vi "Initial AO Voltage.vi"(8 "error in":errorcluster, 11 "AO Properties":T1) -> (0 "error out":errorcluster, 3 "DAQ Ref out":refnum<k21>)   [LabVIEW 2021, in "DAQ Analog InOut Engine.lvlib"]
uses:
  DAQ Analog InOut Engine.lvlib
  AO Properties.ctl
  System Explorer/Types/Output Channel Parameters.ctl
  <vilib>/DAQmx/create/channels.llb/DAQmx Create Channel (AO-Voltage-Basic).vi
  System Explorer/DAQ Analog InOut System Explorer.lvlib
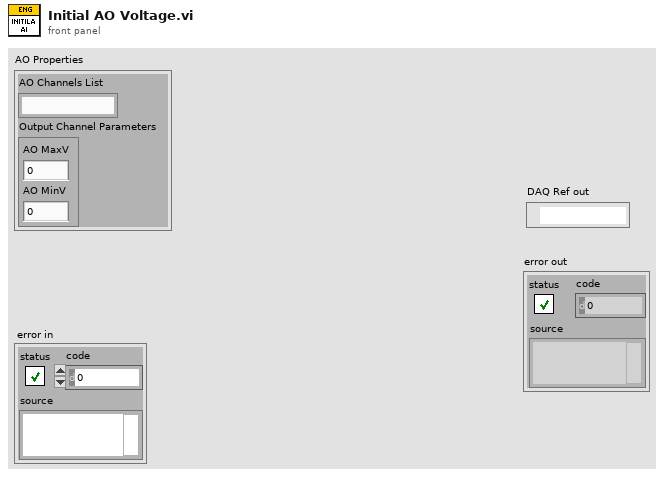
[diagram p1: front panel]
types:
  T1 = typedef "DAQ Analog InOut Engine.lvlib/AO Properties.ctl" = cluster{"AO Channels List":string, "Output Channel Parameters":T2}
  T2 = typedef "DAQ Analog InOut System Explorer.lvlib/Output Channel Parameters.ctl" = cluster{"AO MaxV":dbl, "AO MinV":dbl}
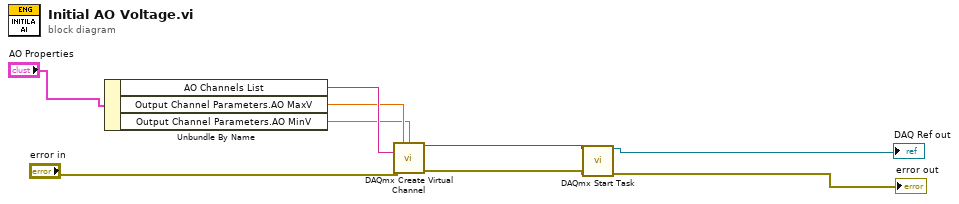
[diagram p0: block diagram]
diagram:
  n1 = Unbundle By Name("AO Properties") -> ("AO Channels List"=w7:string, "Output Channel Parameters.AO MaxV"=w6:dbl, "Output Channel Parameters.AO MinV"=w5:dbl)
  n2 = call-poly <vilib>:"DAQmx Create Virtual Channel.vi"("maximum value"=w6, "minimum value"=w5, "physical channels"=w7, "error in"="error in") -> ("task out"=w4:refnum<k21>, "error out"=w3:errorcluster)  [unwired: 10 in]
  n3 = call <vilib>:"DAQmx Start Task.vi"("task/channels in"=w4, "error in"=w3) -> ("task out"=→"DAQ Ref out":refnum<k21>, "error out"=→"error out":errorcluster)  [unwired: 12 in]
